vi "WriteTestedDB.vi"(8 "error in":errorcluster caption="错误输入", 11 "ParaIn":T1={"DeviceType"="TBOX", "PartNumber"="1805", "TUID"="", "Hw"="Hw", "Sw"="Sw", "PTime"="Sw", "SN"="", "Certid"="", "ICCID"="", "Imei"="", "AuthCode"="", "MAC"="", "Result"=""}) -> (0 "error out":errorcluster caption="错误输出", 3 "ReportStrA":string)   [LabVIEW 2013]
uses:
  DBPara.ctl
panel:
  out "连接的字符串":string
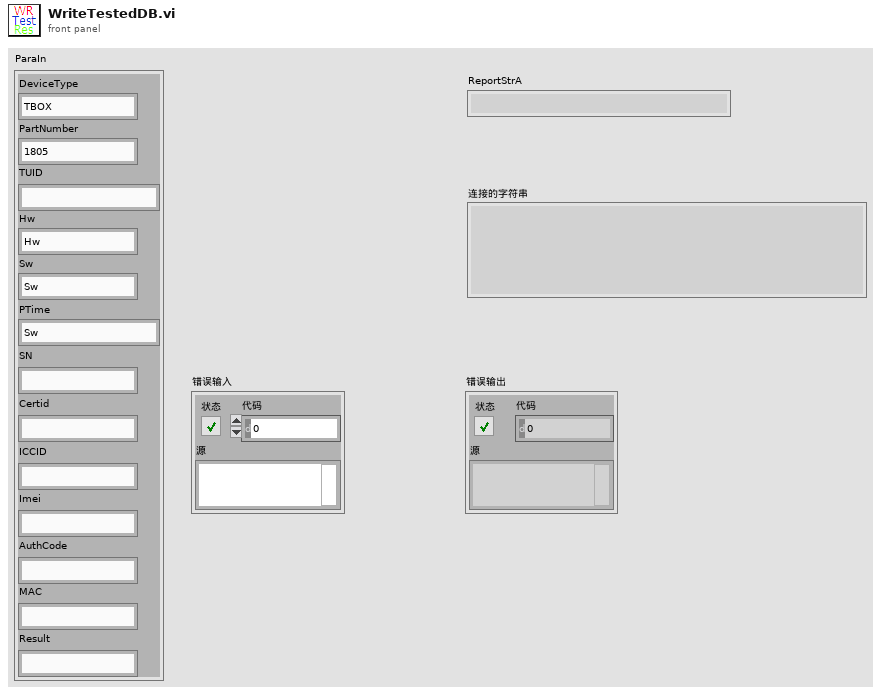
[diagram p1: front panel]
types:
  T1 = typedef "DBPara.ctl" = cluster{"DeviceType":string, "PartNumber":string, "TUID":string, "Hw":string, "Sw":string, "PTime":string, "SN":string, "Certid":string, "ICCID":string, "Imei":string, "AuthCode":string, "MAC":string, "Result":string}
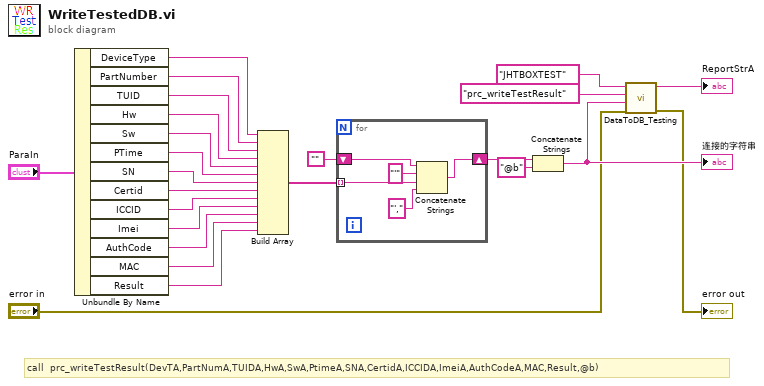
[diagram p0: block diagram]
diagram:
  # "call  prc_writeTestResult(DevTA,PartNumA,TUIDA,HwA,SwA,PtimeA,SNA,CertidA,ICCIDA,ImeiA,AuthCodeA,MAC,Result,@b)"
  n1 = Unbundle By Name("ParaIn") -> ("DeviceType"=w16:string, "PartNumber"=w15:string, "TUID"=w14:string, "Hw"=w13:string, "Sw"=w12:string, "PTime"=w11:string, "SN"=w10:string, "Certid"=w9:string, "ICCID"=w8:string, "Imei"=w7:string, "AuthCode"=w6:string, "MAC"=w5:string, "Result"=w4:string)
  n2 = Build Array(w16, w15, w14, w13, w12, w11, w10, w9, w8, w7, w6, w5, w4) -> (w3:string[])
  n3 = for {
    shift-right: [w28] -> w23
    shift-left: "" -> [w29]
    tunnel: w3 -> [w25] mode=indexing
    n4 = Concatenate Strings(w29, "'", w25, "',") -> (w28:string)
  }
  n5 = Concatenate Strings(w23, "@b") -> (w19:string)
  "连接的字符串" <- w19
  n6 = call "DataToDB_Testing.vi"("error in (no error)"="error in", "all string"=w19, "Procedure name"="prc_writeTestResult", "DSN name"="JHTBOXTEST") -> ("error out"=→"error out":errorcluster, "ReportStrA"=→"ReportStrA":string)  [unwired: 6 in]
